vi "uPolicy_TopicIsRelevant.vi"(8 "error in (no error)":errorcluster, 10 "Observed Topic (Lower Case)":string, 11 "Decorate in":refnum<class "Decorate.lvclass">) -> (0 "error out":errorcluster, 2 "Relevant?":bool, 3 "Decorate out":refnum<class "Decorate.lvclass">)   [LabVIEW 2023, in "uLib.lvlib" / "Decorate.lvclass"]
uses:
  Decorate.lvclass
  Decorate.lvclass/Decorate.ctl
  uPolicy/uPolicy.lvclass
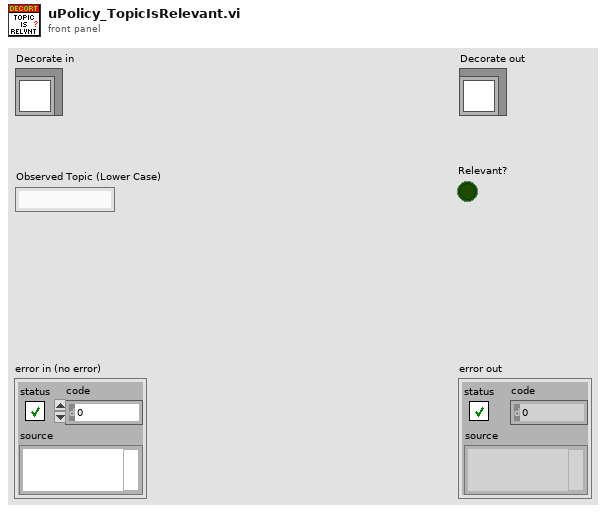
[diagram p1: front panel]
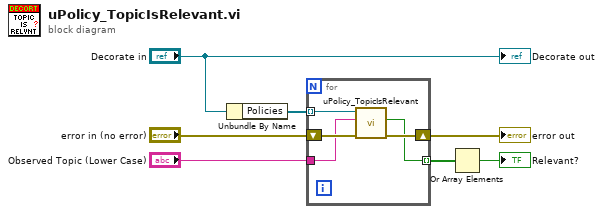
[diagram p0: block diagram]
diagram:
  n1 = Unbundle By Name("Decorate in") -> ("Policies"=w6:refnum<class "uPolicy.lvclass">[])
  n2 = for {
    tunnel: w6 -> [w12] mode=indexing
    shift-right: [w10] -> w4
    shift-left: "error in (no error)" -> [w11]
    tunnel: "Observed Topic (Lower Case)" -> [w9]
    tunnel: [w8] -> w2 mode=indexing
    n3 = call-dynamic "uPolicy_TopicIsRelevant.vi"("error in (no error)"=w11, "Observed Topic (Lower Case)"=w9, "uPolicy_All in"=w12) -> ("error out"=w10:errorcluster, "Relevant?"=w8:bool)  [unwired: 6 in, 1 out]
  }
  "error out" <- w4
  n4 = Or Array Elements(Boolean array=w2) -> (logical OR=→"Relevant?":bool)
  "Decorate out" <- "Decorate in"
